vi "Warp Perspective (Greyscale).vi"(4 "Border Colour (Default: 0)":u8, 5 "Boarder Type (Default: DEFAULT)":T2=enum."DEFAULT", 6 "Required Destination Size":T5, 7 "Interpolation Mode (Default: CUBIC)":T4=enum."CUBIC", 8 "error in (no error)":errorcluster, 9 "3x3 Warp Matrix":T1, 10 "Greyscale Destination Image in":T3, 11 "Greyscale Source Image in":T3) -> (0 "error out":errorcluster, 3 "Greyscale Destination Image":T3)   [LabVIEW 2020, in "image.lvlib"]
doc: "Warp the Source Image based on the 3x3 Warp Matrix.\n\nA Warp Matrix can be computed using the \"Get Perspective Transform.vi\""
uses:
  image.lvlib
  Greyscale Image.ctl
  common/Image Size (Integer).ctl
  Interpolation Mode.ctl
  Border Type.ctl
  <vilib>/Analysis/Matrix/Datatypes/RealMatrix.ctl
  2e2371c9-0103-42e0-a64c-538b92d2b12b.vi
  2e2371c9-0103-42e0-a64c-538b92d2b12b.vi/0c263cf4-9042-4d44-b92e-dafa676e1650.vi
  <vilib>/Utility/error.llb/Error Cluster From Error Code.vi
  common/common.lvlib
  <vilib>/Analysis/Matrix/NI_Matrix.lvlib
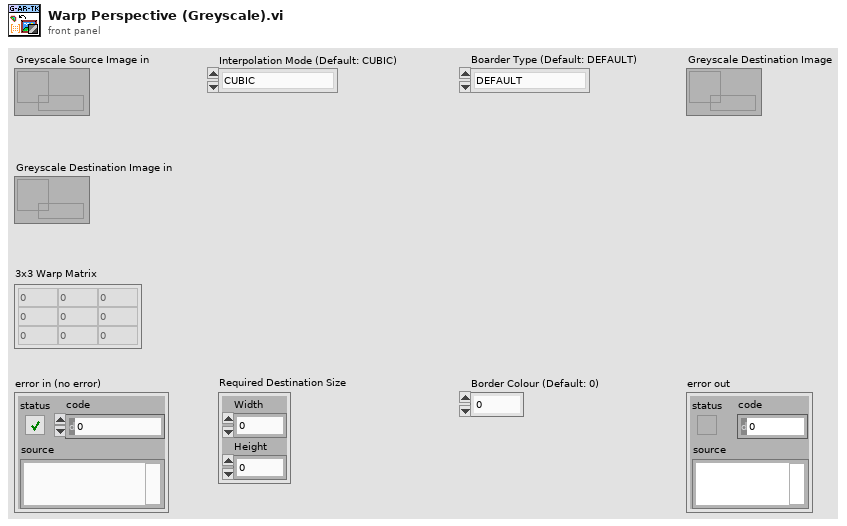
[diagram p1: front panel]
types:
  T1 = typedef "NI_Matrix.lvlib/RealMatrix.ctl" = dbl[][]
  T2 = typedef "image.lvlib/Border Type.ctl" = enum8{"CONSTANT", "REPLICATE", "REFLECT", "WRAP", "TRANSPARENT", "DEFAULT", "ISOLATED"}
  T3 = typedef "image.lvlib/Greyscale Image.ctl" = refnum<data-value>
  T4 = typedef "image.lvlib/Interpolation Mode.ctl" = enum8{"NEAREST", "LINEAR", "CUBIC", "AREA", "LANCZOS", "LINEAR_EXACT", "NEAREST_EXACT", "MAX"}
  T5 = typedef "common.lvlib/Image Size (Integer).ctl" = cluster{"Width":u16, "Height":u16}
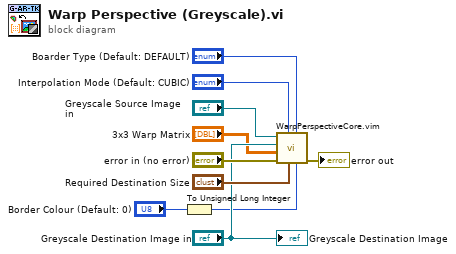
[diagram p0: block diagram]
diagram:
  n1 = To Unsigned Long Integer(number="Border Colour (Default: 0)") -> (unsigned 32bit integer=w1:u32)
  n2 = call "WarpPerspectiveCore.vim"("Border Colour"=w1, "Boarder Type"="Boarder Type (Default: DEFAULT)", "Destination Size"="Required Destination Size", "Interpolation Mode"="Interpolation Mode (Default: CUBIC)", "error in (no error)"="error in (no error)", "Homography"="3x3 Warp Matrix", "Dst"="Greyscale Destination Image in", "Src"="Greyscale Source Image in") -> ("error out"=→"error out":errorcluster)  [unwired: 3 in]
  "Greyscale Destination Image" <- "Greyscale Destination Image in"
